vi "Extend Array.vi"(10 "Extend to size":i32, 11 "Array in":dbl[](array[numeric])) -> (2 "Extended":bool, 3 "Array out":dbl[](array[numeric]))   [LabVIEW 2016]
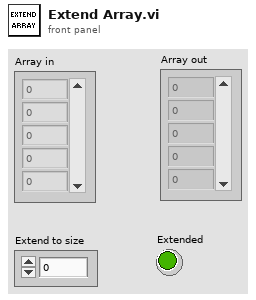
[diagram p1: front panel]
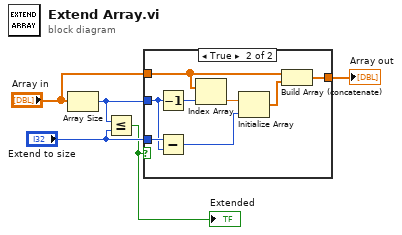
[diagram p0: block diagram]
diagram:
  n1 = Array Size(array="Array in") -> (size(s)=w3:i32)
  n2 = Less Or Equal?(x=w3, y="Extend to size") -> (x <= y?=w1:bool)
  "Extended" <- w1
  n3 = case shown="True" w1 {
    tunnel: "Extend to size" -> [_ w14]
    tunnel: w3 -> [_ w13]
    tunnel: "Array in" -> [w6 w9]
    tunnel: [w6 w7] -> w4
    frame False {
    }
    frame True {
      n4 = Decrement(x=w13) -> (x-1=w12:i32)
      n5 = Subtract(x=w14, y=w13) -> (x-y=w11:i32)
      n6 = Index Array(array=w9, index=w12) -> (element=w10:dbl)
      n7 = Initialize Array(w10, w11) -> (w8:dbl[])
      n8 = Build Array (concatenate)(w9, w8) -> (w7:dbl[])
    }
  }
  "Array out" <- w4
